vi "led blink.vi"(6 "Color Box 2":u32(colorbox)=15663126, 7 "Color Box":u32(colorbox)=3014911, 8 "PWM Channel":T1=enum."PWM 9") -> (5 "LED Strip":u32[](array[colorbox]))   [LabVIEW 2019]
uses:
  <vilib>/Rock Robotics/SystemInterfaces/DIO/FPGA_DIOPWMChannel.ctl
panel:
  in  "String Length":u16=8
  in  "stop":bool
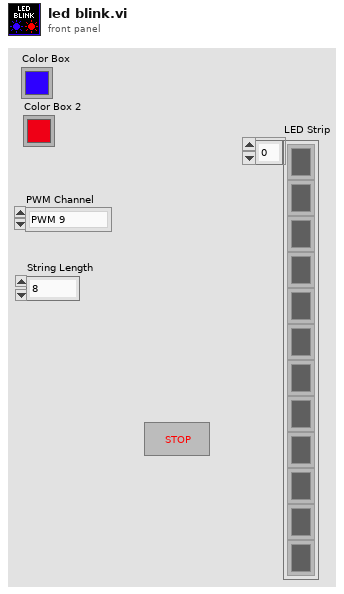
[diagram p1: front panel]
types:
  T1 = typedef "FPGA_DIOPWMChannel.ctl" = enum8{"PWM 0", "PWM 1", "PWM 2", "PWM 3", "PWM 4", "PWM 5", "PWM 6", "PWM 7", "PWM 8", "PWM 9", "PWM MXP 0", "PWM MXP 1", "PWM MXP 2", "PWM MXP 3", "PWM MXP 4", "PWM MXP 5", "PWM MXP 6", "PWM MXP 7", "PWM MXP 8", "PWM MXP 9", "Invalid"}
  T2 = typedef "WPI_PWMDeviceRef.ctl" = cluster{"DeviceStatus":errorcluster, "PWM Channel":T1}
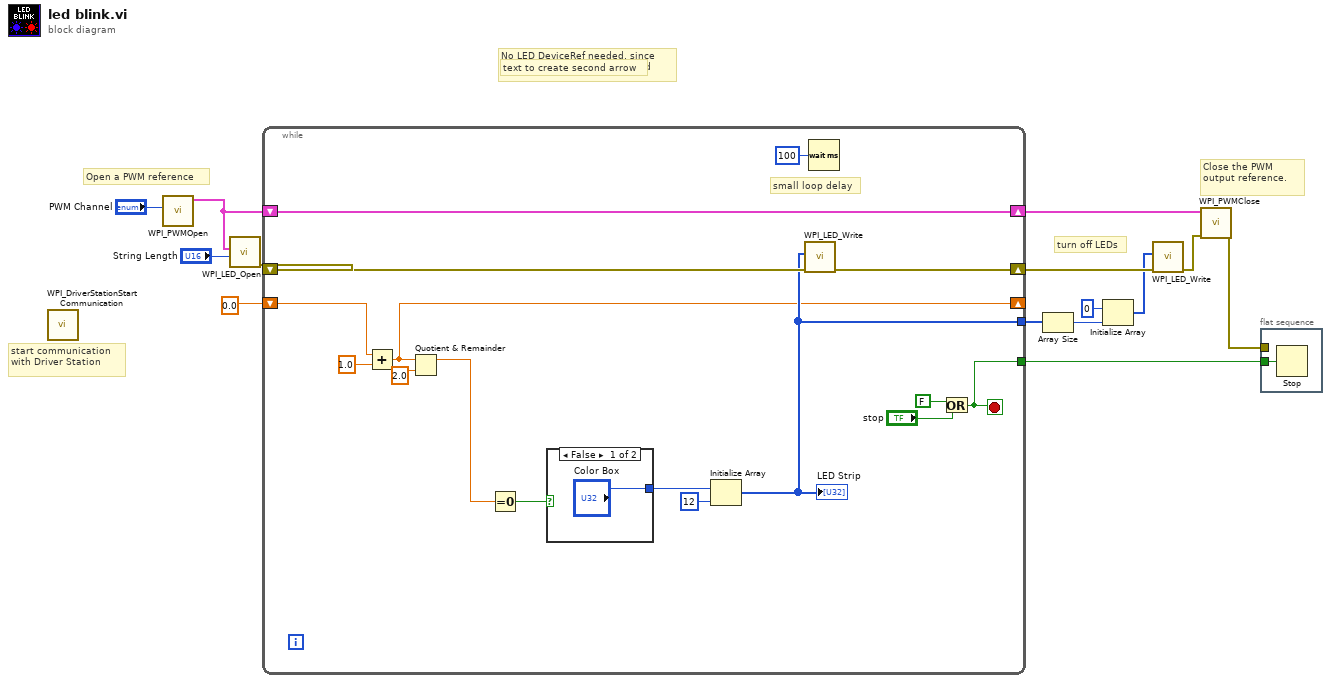
[diagram p0: block diagram]
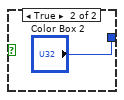
[diagram p2: hidden frame]
diagram:
  # "Open a PWM reference"
  # "start communication with Driver Station"
  # "turn off LEDs"
  # "No LED DeviceRef needed, since only one LED strip is supported"
  # "Close the PWM output reference."
  # "text to create second arrow"
  n1 = call <vilib>:"WPI_DriverStationStart Communication.vi"() -> ()  [unwired: 2 in, 10 out]
  n2 = call <vilib>:"WPI_PWMOpen.vi"("PWM Channel"="PWM Channel") -> ("PWMDeviceRef"=w2:T2)  [unwired: 9 in, 1 out]
  n3 = call <vilib>:"WPI_LED_Open.vi"("String Length"="String Length", "PWMDeviceRef"=w2) -> ("error out"=w12:errorcluster)  [unwired: 9 in]
  n4 = while {
    shift-right: [w27] -> w13
    shift-left: w2 -> [w27]
    tunnel: [w29] -> w14
    shift-right: [w25] -> w11
    shift-left: w12 -> [w26]
    tunnel: [w24] -> w8
    shift-right: [w19] -> _
    shift-left: 0.0 -> [w20]
    stop <- w29 stop-if-true
    # "small loop delay"
    n5 = Add(x=w20, y=1.0) -> (x+y=w19:dbl)
    n6 = Quotient & Remainder(x=w19, y=2.0) -> (x-y*floor(x/y)=w16:dbl)  [unwired: 1 out]
    n7 = Equal To 0?(x=w16) -> (x = 0?=w17:bool)
    n8 = case shown="False" w17 {
      tunnel: ["Color Box" "Color Box 2"] -> w23
      frame False {
      }
      frame True {
      }
    }
    n9 = Initialize Array(w23, 12 ("dimension size")) -> (w24:u32[])
    "LED Strip" <- w24
    n10 = call <vilib>:"WPI_LED_Write.vi"("error in"=w26, "Color Array"=w24) -> ("error out"=w25:errorcluster)  [unwired: 9 in]
    n11 = Wait (ms)(milliseconds to wait=u32 100) -> ()  [unwired: 1 out]
    n12 = Or(x=FALSE, y="stop") -> (x .or. y?=w29:bool)
  }
  n13 = Array Size(array=w8) -> (size(s)=w9:i32)
  n14 = Initialize Array(u32 0, w9) -> (w6:u32[])
  n15 = call <vilib>:"WPI_LED_Write.vi"("error in"=w11, "Color Array"=w6) -> ("error out"=w10:errorcluster)  [unwired: 9 in]
  n16 = call <vilib>:"WPI_PWMClose.vi"("error in (no error)"=w10, "PWMDeviceRef"=w13) -> ("error out"=w5:errorcluster)  [unwired: 9 in]
  n17 = flat-sequence {
    tunnel: w14 -> [w33]
    tunnel: w5 -> [_]
    frame #0 {
      n18 = Stop(stop? (T)=w33) -> ()
    }
  }
